vi "nominal ingest tabular set timestamp relative.vi"(6 "has_offset":bool, 7 "offset_ms":dbl, 8 "error in (no error)":errorcluster, 9 "time_unit":i32, 10 "column":string, 11 "staging":i32) -> (0 "error out":errorcluster, 3 "function return":i32)   [LabVIEW 2020, in "client.lvlib"]
doc: "int32_t nominal_ingest_tabular_set_timestamp_relative(int32_t staging,\n const char *column,\n int32_t time_unit,\n double offset_ms,\n bool has_offset);"
uses:
  client.lvlib
  bin/nominalClient_64.dll
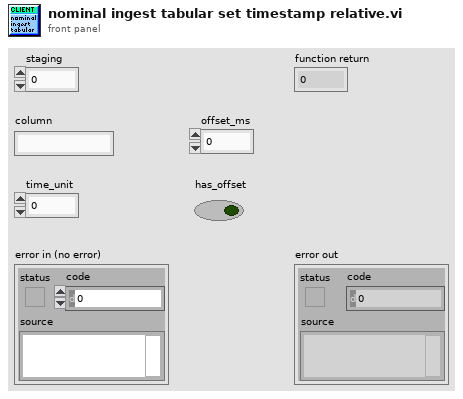
[diagram p1: front panel]
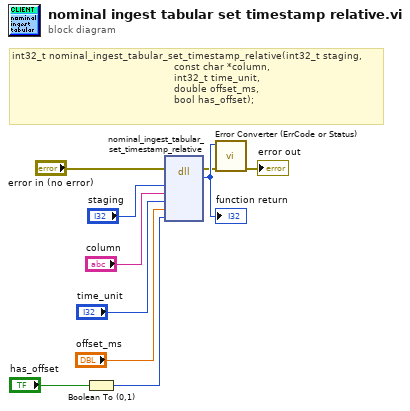
[diagram p0: block diagram]
diagram:
  # "int32_t nominal_ingest_tabular_set_timestamp_relative(int32_t staging,\n                                                      const char *column,\n                                                      int32_t time_unit,\n                                                      double offset_ms,\n                                                      bool has_offset);"
  n1 = Boolean To (0,1)(Boolean="has_offset") -> (0, 1=w4:i16)
  n2 = dll-call lib="C:/code/labview-client-rs/lv_src/bin/nominalClient_*.*" fn="nominal_ingest_tabular_set_timestamp_relative"(error in="error in (no error)", "staging"="staging", "column"="column", "time_unit"="time_unit", "offset_ms"="offset_ms", "has_offset"=w4) -> (error out=w2:errorcluster, w10:i32)  [unwired: 7 in, 1 out]
  "function return" <- w10
  n3 = call "Error Converter (ErrCode or Status).vi"("error in (no error)"=w2, "error code"=w10) -> ("error out"=→"error out":errorcluster)  [unwired: 9 in]
